vi "MWIR.vi"(4 "error in (no error)":errorcluster, 6 "current":dbl, 7 "connection ID":refnum<k5>) -> (0 "error out":errorcluster, 3 "connection ID out":refnum<k5>)   [LabVIEW 2025, in "CAENels FAST-PS.lvlib"]
doc: "The MWIR block is used to perform a ramp to the given current setpoint. The use of this command is alternative to the MWI command. The default value of the current slew-rate is stored in the parameter table. To dynamically change the slew-rate value it is possible to use the MSRI Command."
uses:
  CAENels FAST-PS.lvlib
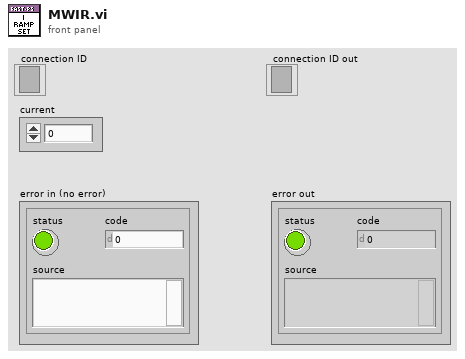
[diagram p1: front panel]
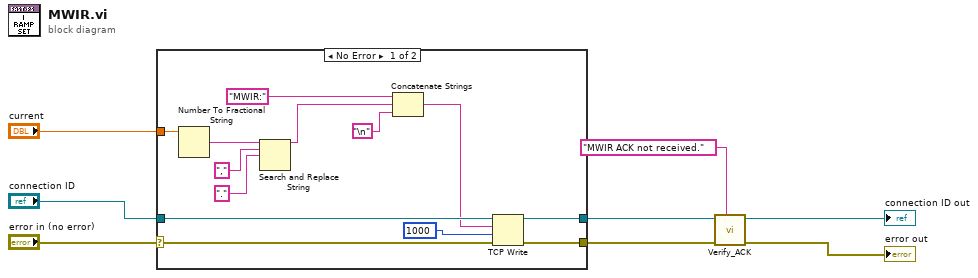
[diagram p0: block diagram]
diagram:
  n1 = case shown="No Error" "error in (no error)" {
    selector: "error in (no error)" -> [w21 w23]
    tunnel: [w20 w23] -> w6
    tunnel: [w19 w22] -> w4
    tunnel: "connection ID" -> [w18 w22]
    tunnel: "current" -> [w11 _]
    frame No Error {
      n2 = Number To Fractional String(number=w11) -> (F-format string=w10:string)  [unwired: 3 in]
      n3 = Search and Replace String(input string=w10, search string=",", replace string=".") -> (result string=w14:string)  [unwired: 5 in, 3 out]
      n4 = Concatenate Strings("MWIR:" ("string (\"\")"), w14, "\n") -> (w16:string)
      n5 = TCP Write(connection ID=w18, data in=w16, error in (no error)=w21, 9:1000 ("timeout ms (25000)")) -> (connection ID out=w19:refnum<k5>, error out=w20:errorcluster)  [unwired: 1 out]
    }
    frame Error {
    }
  }
  n6 = call "Verify_ACK.vi"("error code description"="MWIR ACK not received.", "error in (no error)"=w6, "connection ID"=w4) -> ("error out"=→"error out":errorcluster, "connection ID out"=→"connection ID out":refnum<k5>)  [unwired: 5 in]
